vi "aimingPID.vi"(8 "bias":dbl, 9 "Kp":dbl, 10 "setpoint":dbl, 11 "process variable":dbl) -> (0 "error":dbl, 3 "output":dbl)   [LabVIEW 2016]
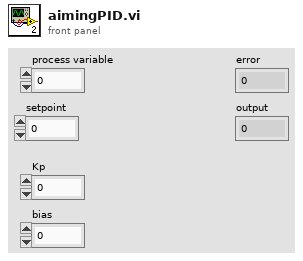
[diagram p1: front panel]
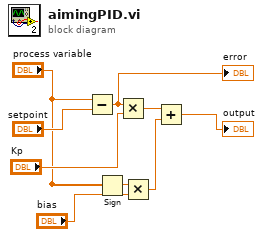
[diagram p0: block diagram]
diagram:
  n1 = Subtract(x="process variable", y="setpoint") -> (x-y=w7:dbl)
  "error" <- w7
  n2 = Sign(1:"process variable") -> ()  [unwired: 1 out]
  n3 = Multiply(x=w7, y="Kp") -> (x*y=w5:dbl)
  n4 = Multiply(x="process variable", y="bias") -> (x*y=w1:dbl)
  n5 = Add(x=w5, y=w1) -> (x+y=→"output":dbl)
